vi "Turn 2.vi"(9 "Range of accuracy":sgl, 10 "desired angle":sgl) -> (1 "In Range?":bool, 2 "coerced(x)":dbl)   [LabVIEW 2020]
uses:
  Robot Global Data.vi
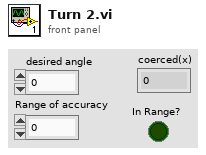
[diagram p1: front panel]
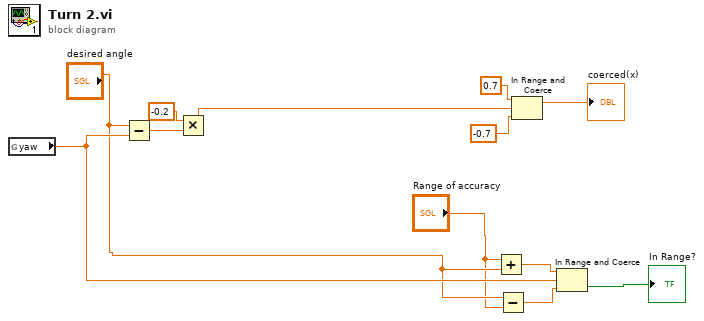
[diagram p0: block diagram]
diagram:
  n1 = global read "Robot Global Data.vi" "yaw"() -> (w9:dbl)
  n2 = Subtract(x="desired angle", y=w9) -> (x-y=w5:dbl)
  n3 = Multiply(x=-0.2, y=w5) -> (x*y=w4:dbl)
  n4 = Add(x="Range of accuracy", y="desired angle") -> (x+y=w11:sgl)
  n5 = Subtract(x="desired angle", y="Range of accuracy") -> (x-y=w10:sgl)
  n6 = In Range and Coerce(upper limit=0.7, x=w4, lower limit=-0.7) -> (coerced(x)=→"coerced(x)":dbl)  [unwired: 1 out]
  n7 = In Range and Coerce(upper limit=w11, x=w9, lower limit=w10) -> (In Range?=→"In Range?":bool)  [unwired: 1 out]
